vi "eFGV - Generated Error.vi"(6 "eFGV States":T1, 8 "Error In":errorcluster, 10 "State":string, 11 "This VI":refnum<vi>) -> (0 "Error Out":errorcluster, 2 "Event Generated Error":refnum<user-event>)   [LabVIEW 2020]
uses:
  Control/State - eFGV.ctl
  Control/Error Info.ctl
  <vilib>/Utility/error.llb/DialogType.ctl
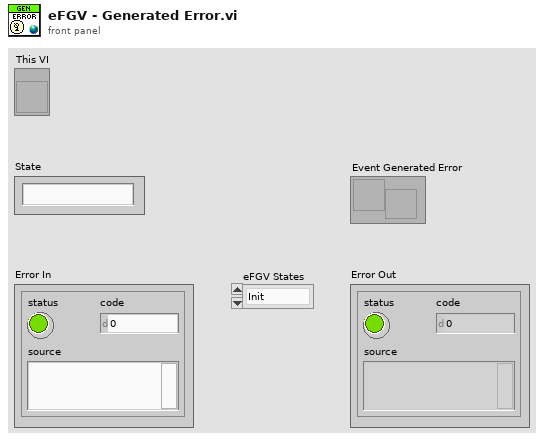
[diagram p1: front panel]
types:
  T1 = typedef "State - eFGV.ctl" = enum16{"Init", "Read", "Write", "Exit"}
  T2 = typedef "Error Info.ctl" = cluster{"Date":string, "Time":string, "Code":string, "VI Name":string, "State":string, "Message":string}
  T3 = typedef "DialogType.ctl" = u16
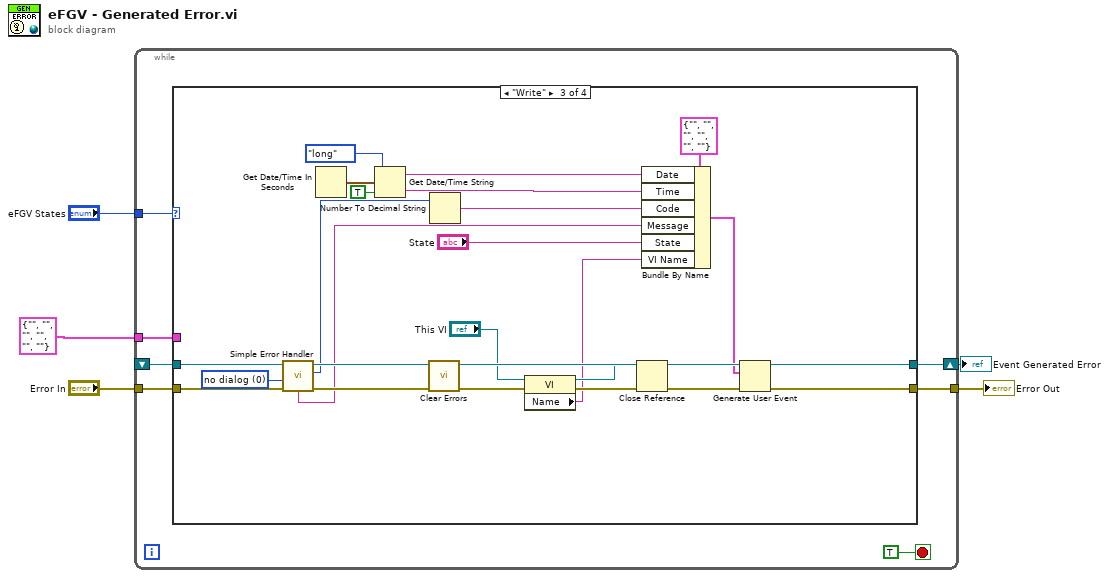
[diagram p0: block diagram]
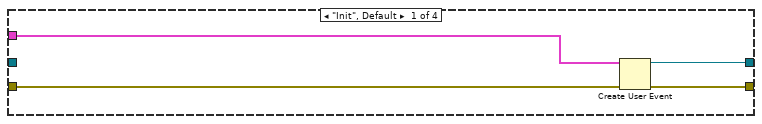
[diagram p2: hidden frame]
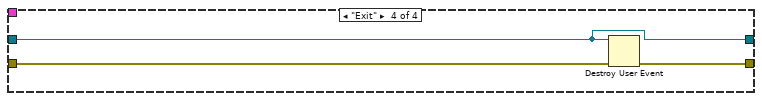
[diagram p4: hidden frame]
diagram:
  n1 = while {
    tunnel: "Error In" -> [w12]
    tunnel: [w11] -> w5
    tunnel: "eFGV States" -> [w9]
    tunnel: T2 {"Date"="", "Time"="", "Code"="", "VI Name"="", "State"="", "Message"=""} ("Error Status") -> [w8]
    shift-right: [w7] -> w1
    shift-left: _ -> [w6]
    stop <- TRUE stop-if-true
    n2 = case shown="\"Write\"" w9 {
      tunnel: w12 -> [w16 w18 w37 w44]
      tunnel: [w15 w18 w41 w43] -> w11
      tunnel: w8 -> [w13 _ _ _]
      tunnel: [w14 w17 w34 w42] -> w7
      tunnel: w6 -> [_ w17 w35 w42]
      frame "Init", Default {
        n3 = Create User Event(user event datatype=w13, error in=w16) -> (user event=w14:refnum<user-event>, error out=w15:errorcluster)
      }
      frame "Read" {
      }
      frame "Write" {
        w24 = T3 0 items=["no dialog", "OK message", "continue or stop message", "OK message + warnings", "continue/stop + warnings"] ("type of dialog (OK msg:1)")
        n4 = call <vilib>:"Simple Error Handler.vi"("type of dialog (OK msg:1)"=w24, "error in (no error)"=w37) -> ("code out"=w25:i32, "error out"=w36:errorcluster, "message"=w23:string)  [unwired: 3 in, 2 out]
        n5 = Get Date/Time In Seconds() -> (seconds since 1Jan1904=w31:timestamp)
        n6 = Get Date/Time String(date format (0)=enum16{"short", "long", "abbreviated"}."long", seconds (now)=w31, want seconds? (F)=TRUE) -> (date string=w26:string, time string=w27:string)
        n7 = call <vilib>:"Clear Errors.vi"("error in (no error)"=w36) -> ("error out"=w39:errorcluster)  [unwired: 5 in, 1 out]
        n8 = Number To Decimal String(number=w25) -> (decimal integer string=w28:string)  [unwired: 1 in]
        n9 = property class="VI"(reference="This VI", error in=w39) -> (reference out=w33:refnum<vi>, error out=w40:errorcluster, "Name"=w21:string)
        n10 = Close Reference(reference=w33, error in (no error)=w40) -> (error out=w38:errorcluster)
        n11 = Bundle By Name(cluster=T2 {"Date"="", "Time"="", "Code"="", "VI Name"="", "State"="", "Message"=""} ("Error Status"), "Date"=w26, "Time"=w27, "Code"=w28, "Message"=w23, "State"="State", "VI Name"=w21) -> (w22:T2)
        n12 = Generate User Event(user event=w35, event data cluster=w22, error in=w38) -> (user event out=w34:refnum<user-event>, error out=w41:errorcluster)  [unwired: 1 in]
      }
      frame "Exit" {
        n13 = Destroy User Event(user event=w42, error in=w44) -> (error out=w43:errorcluster)
      }
    }
  }
  "Error Out" <- w5
  "Event Generated Error" <- w1
